vi "Lang Set Tab.vi"(8 "error in (no error)":errorcluster, 10 "Tab":T1, 11 "Configuration Window in":refnum<class "Configuration Window.lvclass">) -> (0 "error out":errorcluster, 3 "Configuration Window out":refnum<class "Configuration Window.lvclass">)   [LabVIEW 2018, in "Configuration Window.lvlib" / "Configuration Window.lvclass"]
uses:
  Configuration Window.lvclass
  Framework/Framework/Const Lang Property.ctl
  Framework/Framework/Framework.lvclass
  Framework/Framework/Const Lang CfgWnd Tab.ctl
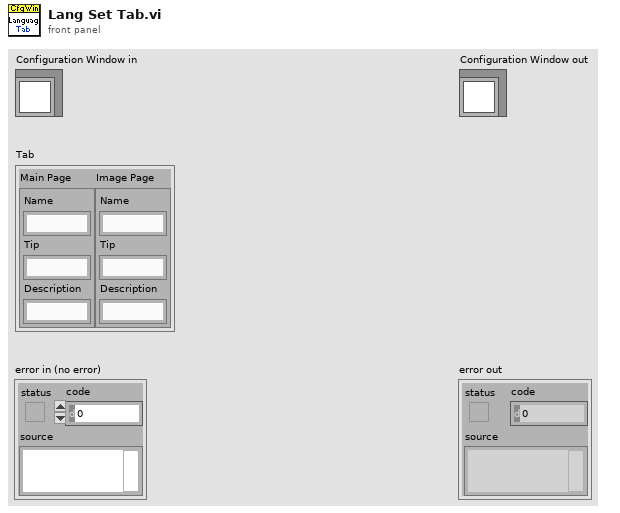
[diagram p1: front panel]
types:
  T1 = typedef "Framework.lvlib/Framework.lvclass/Const Lang CfgWnd Tab.ctl" = cluster{"Main Page":T2, "Image Page":T2}
  T2 = typedef "Framework.lvlib/Framework.lvclass/Const Lang Property.ctl" = cluster{"Name":string, "Tip":string, "Description":string}
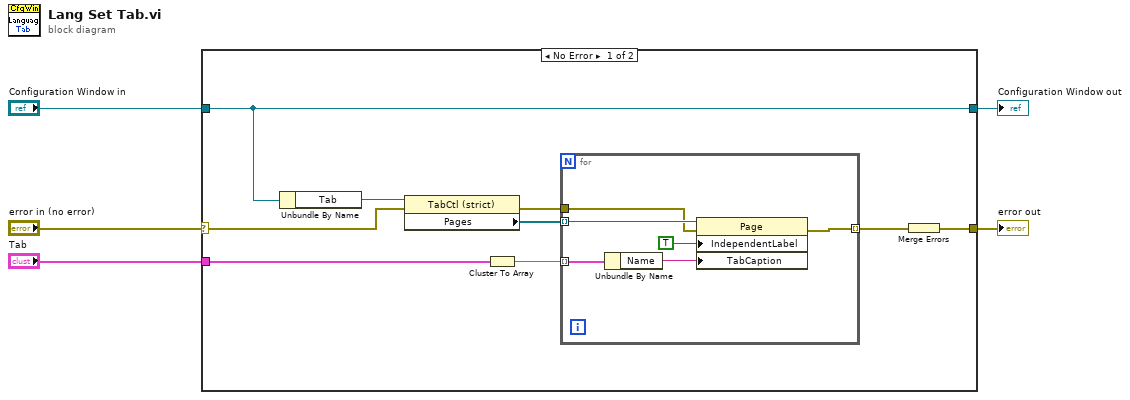
[diagram p0: block diagram]
diagram:
  n1 = case shown="No Error" "error in (no error)" {
    selector: "error in (no error)" -> [w9 w22]
    tunnel: [w6 w22] -> w4
    tunnel: [w13 w21] -> w2
    tunnel: "Configuration Window in" -> [w13 w21]
    tunnel: "Tab" -> [w10 _]
    frame No Error {
      n2 = Unbundle By Name(w13) -> ("Tab"=w12:refnum<vi>)
      n3 = property class="TabCtl (strict)"(reference=w12, error in=w9) -> (error out=w8:errorcluster, "Pages"=w11:refnum<vi>[])  [unwired: 1 out]
      n4 = Cluster To Array(cluster=w10) -> (array=w14:T2[])
      n5 = for {
        tunnel: w14 -> [w18] mode=indexing
        tunnel: w11 -> [w20] mode=indexing
        tunnel: [w16] -> w7 mode=indexing
        tunnel: w8 -> [w15]
        n6 = Unbundle By Name(w18) -> ("Name"=w17:string)
        n7 = property class="Page"(reference=w20, error in=w15, "IndependentLabel"=TRUE ("Independent Label"), "TabCaption"=w17) -> (error out=w16:errorcluster)  [unwired: 1 out]
      }
      n8 = Merge Errors(w7) -> (w6:errorcluster)
    }
    frame Error {
    }
  }
  "error out" <- w4
  "Configuration Window out" <- w2
